vi "Configure Impedance.vi"(8 "error in (no error)":errorcluster, 10 "Output Impedance (50 Ohm)":i32=50, 11 "VISA resource name":refnum<visa-resource-name>) -> (0 "error out":errorcluster, 3 "VISA resource name out":refnum<visa-resource-name>)   [LabVIEW 2012, in "Fluke 5080.lvlib"]
doc: "Configures the impedance used for dBm outputs."
uses:
  <instrlib>/Fluke 5080/Fluke 5080.lvlib
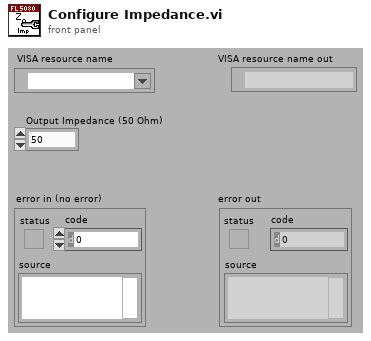
[diagram p1: front panel]
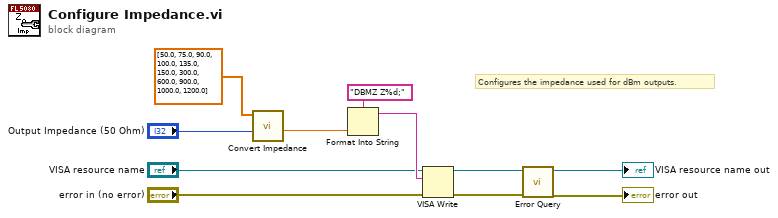
[diagram p0: block diagram]
diagram:
  # "Configures the impedance used for dBm outputs."
  n1 = call <instrlib>:"Convert Impedance.vi"("Input Impedance (0 Ohm)"="Output Impedance (50 Ohm)", "Discrete Value List"=dbl[] [50.0, 75.0, 90.0, 100.0, 135.0, 150.0, 300.0, 600.0, 900.0, 1000.0, 1200.0]) -> ("Output Impedance"=w2:dbl)  [unwired: 9 out]
  n2 = Format Into String(format string="DBMZ Z%d;", w2) -> (resulting string=w10:string)  [unwired: 2 in, 1 out]
  n3 = VISA Write(VISA resource name="VISA resource name", write buffer=w10, error in (no error)="error in (no error)") -> (VISA resource name out=w7:refnum<visa-resource-name>, error out=w6:errorcluster)  [unwired: 1 out]
  n4 = call <instrlib>:"Error Query.vi"("error in (no error)"=w6, "VISA resource name"=w7) -> ("error out"=→"error out":errorcluster, "VISA resource name out"=→"VISA resource name out":refnum<visa-resource-name>)  [unwired: 8 out]
